vi "Bus Parameters to String.vi"(0 "Bus":T1={"Name"="", "Bus_Number"=0, "Bus_Controller"={"BC_Messages"=[{"Name"="Gun_One", "Tx-Rx_T-Tx"=FALSE, "RT_Address"=11, "RT_SA_Address"=10, "Parameters"=[{"name"="Data_01", "firstByte"=8, "startBit"=0, "numberBits"=8, "scaleFactor"=1.0, "scaleOffset"=0.0, "signed"=FALSE}], "Transfer Enabled"=TRUE, "Message Buffer ID"=0, "Default_Message_Buffer_Data"=[0, 1, 2, 3, 4, 5, 6, 7, 8, 9, 10, 11, 12, 13, 14, 15, 16, 17, 18, 19, 20, 21, 22, 23, 24, 25, 26, 27, 28, 29], "Word_Count"=30}, {"Name"="Gun_Two", "Tx-Rx_T-Tx"=FALSE, "RT_Address"=11, "RT_SA_Address"=5, "Parameters"=[{"name"="Data_02", "firstByte"=8, "startBit"=0, "numberBits"=8, "scaleFactor"=1.0, "scaleOffset"=0.0, "signed"=FALSE}], "Transfer Enabled"=TRUE, "Message Buffer ID"=1, "Default_Message_Buffer_Data"=[0, 5, 10, 15, 20, 25, 30, 35, 40, 45, 50, 55, 60, 65, 70, 75, 80, 85, 90, 95, 100, 105, 110, 115, 120, 125, 130, 135, 140, 145], "Word_Count"=30}, {"Name"="Get_It", "Tx-Rx_T-Tx"=TRUE, "RT_Address"=5, "RT_SA_Address"=4, "Parameters"=[{"name"="Data_00", "firstByte"=1, "startBit"=0, "numberBits"=8, "scaleFactor"=1.0, "scaleOffset"=0.0, "signed"=FALSE}], "Transfer Enabled"=TRUE, "Message Buffer ID"=2, "Default_Message_Buffer_Data"=[0, 25, 50, 75, 100, 125, 150, 175, 200, 225, 250, 275, 300, 325, 350, 375, 400, 425, 450, 475, 500, 525, 550, 575, 600, 625, 650, 675, 700, 725], "Word_Count"=30}], "Acyclic_Frames"=[], "Enabled"=FALSE}, "Bus_Monitor"={"Name"="", "BM_Messages"=[{"RT_Address"=5, "RT_SubAddress"=1, "Tx-Rx_T-Tx"=TRUE, "Parameters"=[], "Name"=""}, {"RT_Address"=5, "RT_SubAddress"=2, "Tx-Rx_T-Tx"=TRUE, "Parameters"=[], "Name"=""}, {"RT_Address"=5, "RT_SubAddress"=3, "Tx-Rx_T-Tx"=TRUE, "Parameters"=[], "Name"=""}, {"RT_Address"=5, "RT_SubAddress"=4, "Tx-Rx_T-Tx"=TRUE, "Parameters"=[{"name"="BM_Data_Parm_1", "firstByte"=1, "startBit"=0, "numberBits"=8, "scaleFactor"=1.0, "scaleOffset"=0.0, "signed"=FALSE}], "Name"=""}, {"RT_Address"=5, "RT_SubAddress"=5, "Tx-Rx_T-Tx"=TRUE, "Parameters"=[], "Name"=""}, {"RT_Address"=5, "RT_SubAddress"=6, "Tx-Rx_T-Tx"=TRUE, "Parameters"=[], "Name"=""}, {"RT_Address"=5, "RT_SubAddress"=7, "Tx-Rx_T-Tx"=TRUE, "Parameters"=[], "Name"=""}, {"RT_Address"=5, "RT_SubAddress"=8, "Tx-Rx_T-Tx"=TRUE, "Parameters"=[], "Name"=""}, {"RT_Address"=5, "RT_SubAddress"=9, "Tx-Rx_T-Tx"=TRUE, "Parameters"=[], "Name"=""}, {"RT_Address"=5, "RT_SubAddress"=10, "Tx-Rx_T-Tx"=TRUE, "Parameters"=[], "Name"=""}, {"RT_Address"=5, "RT_SubAddress"=11, "Tx-Rx_T-Tx"=TRUE, "Parameters"=[], "Name"=""}, {"RT_Address"=5, "RT_SubAddress"=12, "Tx-Rx_T-Tx"=TRUE, "Parameters"=[], "Name"=""}, {"RT_Address"=5, "RT_SubAddress"=13, "Tx-Rx_T-Tx"=TRUE, "Parameters"=[], "Name"=""}, {"RT_Address"=5, "RT_SubAddress"=14, "Tx-Rx_T-Tx"=TRUE, "Parameters"=[], "Name"=""}, {"RT_Address"=5, "RT_SubAddress"=15, "Tx-Rx_T-Tx"=TRUE, "Parameters"=[], "Name"=""}, {"RT_Address"=5, "RT_SubAddress"=16, "Tx-Rx_T-Tx"=TRUE, "Parameters"=[], "Name"=""}, {"RT_Address"=5, "RT_SubAddress"=17, "Tx-Rx_T-Tx"=TRUE, "Parameters"=[], "Name"=""}, {"RT_Address"=5, "RT_SubAddress"=18, "Tx-Rx_T-Tx"=TRUE, "Parameters"=[], "Name"=""}, {"RT_Address"=5, "RT_SubAddress"=19, "Tx-Rx_T-Tx"=TRUE, "Parameters"=[], "Name"=""}, {"RT_Address"=5, "RT_SubAddress"=20, "Tx-Rx_T-Tx"=TRUE, "Parameters"=[], "Name"=""}, {"RT_Address"=5, "RT_SubAddress"=21, "Tx-Rx_T-Tx"=TRUE, "Parameters"=[], "Name"=""}, {"RT_Address"=5, "RT_SubAddress"=22, "Tx-Rx_T-Tx"=TRUE, "Parameters"=[], "Name"=""}, {"RT_Address"=5, "RT_SubAddress"=23, "Tx-Rx_T-Tx"=TRUE, "Parameters"=[], "Name"=""}, {"RT_Address"=5, "RT_SubAddress"=24, "Tx-Rx_T-Tx"=TRUE, "Parameters"=[], "Name"=""}, {"RT_Address"=5, "RT_SubAddress"=25, "Tx-Rx_T-Tx"=TRUE, "Parameters"=[], "Name"=""}, {"RT_Address"=5, "RT_SubAddress"=26, "Tx-Rx_T-Tx"=TRUE, "Parameters"=[], "Name"=""}, {"RT_Address"=5, "RT_SubAddress"=27, "Tx-Rx_T-Tx"=TRUE, "Parameters"=[], "Name"=""}, {"RT_Address"=5, "RT_SubAddress"=28, "Tx-Rx_T-Tx"=TRUE, "Parameters"=[], "Name"=""}, {"RT_Address"=5, "RT_SubAddress"=29, "Tx-Rx_T-Tx"=TRUE, "Parameters"=[], "Name"=""}, {"RT_Address"=5, "RT_SubAddress"=30, "Tx-Rx_T-Tx"=TRUE, "Parameters"=[], "Name"=""}, {"RT_Address"=5, "RT_SubAddress"=31, "Tx-Rx_T-Tx"=TRUE, "Parameters"=[], "Name"=""}, {"RT_Address"=11, "RT_SubAddress"=1, "Tx-Rx_T-Tx"=TRUE, "Parameters"=[], "Name"=""}, {"RT_Address"=11, "RT_SubAddress"=2, "Tx-Rx_T-Tx"=TRUE, "Parameters"=[], "Name"=""}, {"RT_Address"=11, "RT_SubAddress"=3, "Tx-Rx_T-Tx"=TRUE, "Parameters"=[], "Name"=""}, {"RT_Address"=11, "RT_SubAddress"=4, "Tx-Rx_T-Tx"=TRUE, "Parameters"=[], "Name"=""}, {"RT_Address"=11, "RT_SubAddress"=5, "Tx-Rx_T-Tx"=TRUE, "Parameters"=[], "Name"=""}, {"RT_Address"=11, "RT_SubAddress"=6, "Tx-Rx_T-Tx"=TRUE, "Parameters"=[], "Name"=""}, {"RT_Address"=11, "RT_SubAddress"=7, "Tx-Rx_T-Tx"=TRUE, "Parameters"=[], "Name"=""}, {"RT_Address"=11, "RT_SubAddress"=8, "Tx-Rx_T-Tx"=TRUE, "Parameters"=[], "Name"=""}, {"RT_Address"=11, "RT_SubAddress"=9, "Tx-Rx_T-Tx"=TRUE, "Parameters"=[], "Name"=""}, {"RT_Address"=11, "RT_SubAddress"=10, "Tx-Rx_T-Tx"=TRUE, "Parameters"=[], "Name"=""}, {"RT_Address"=11, "RT_SubAddress"=11, "Tx-Rx_T-Tx"=TRUE, "Parameters"=[], "Name"=""}, {"RT_Address"=11, "RT_SubAddress"=12, "Tx-Rx_T-Tx"=TRUE, "Parameters"=[], "Name"=""}, {"RT_Address"=11, "RT_SubAddress"=13, "Tx-Rx_T-Tx"=TRUE, "Parameters"=[], "Name"=""}, {"RT_Address"=11, "RT_SubAddress"=14, "Tx-Rx_T-Tx"=TRUE, "Parameters"=[], "Name"=""}, {"RT_Address"=11, "RT_SubAddress"=15, "Tx-Rx_T-Tx"=TRUE, "Parameters"=[], "Name"=""}, {"RT_Address"=11, "RT_SubAddress"=16, "Tx-Rx_T-Tx"=TRUE, "Parameters"=[], "Name"=""}, {"RT_Address"=11, "RT_SubAddress"=17, "Tx-Rx_T-Tx"=TRUE, "Parameters"=[], "Name"=""}, {"RT_Address"=11, "RT_SubAddress"=18, "Tx-Rx_T-Tx"=TRUE, "Parameters"=[], "Name"=""}, {"RT_Address"=11, "RT_SubAddress"=19, "Tx-Rx_T-Tx"=TRUE, "Parameters"=[], "Name"=""}, {"RT_Address"=11, "RT_SubAddress"=20, "Tx-Rx_T-Tx"=TRUE, "Parameters"=[], "Name"=""}, {"RT_Address"=11, "RT_SubAddress"=21, "Tx-Rx_T-Tx"=TRUE, "Parameters"=[], "Name"=""}, {"RT_Address"=11, "RT_SubAddress"=22, "Tx-Rx_T-Tx"=TRUE, "Parameters"=[], "Name"=""}, {"RT_Address"=11, "RT_SubAddress"=23, "Tx-Rx_T-Tx"=TRUE, "Parameters"=[], "Name"=""}, {"RT_Address"=11, "RT_SubAddress"=24, "Tx-Rx_T-Tx"=TRUE, "Parameters"=[], "Name"=""}, {"RT_Address"=11, "RT_SubAddress"=25, "Tx-Rx_T-Tx"=TRUE, "Parameters"=[], "Name"=""}, {"RT_Address"=11, "RT_SubAddress"=26, "Tx-Rx_T-Tx"=TRUE, "Parameters"=[], "Name"=""}, {"RT_Address"=11, "RT_SubAddress"=27, "Tx-Rx_T-Tx"=TRUE, "Parameters"=[], "Name"=""}, {"RT_Address"=11, "RT_SubAddress"=28, "Tx-Rx_T-Tx"=TRUE, "Parameters"=[], "Name"=""}, {"RT_Address"=11, "RT_SubAddress"=29, "Tx-Rx_T-Tx"=TRUE, "Parameters"=[], "Name"=""}, {"RT_Address"=11, "RT_SubAddress"=30, "Tx-Rx_T-Tx"=TRUE, "Parameters"=[], "Name"=""}, {"RT_Address"=11, "RT_SubAddress"=31, "Tx-Rx_T-Tx"=TRUE, "Parameters"=[], "Name"=""}, {"RT_Address"=5, "RT_SubAddress"=1, "Tx-Rx_T-Tx"=FALSE, "Parameters"=[], "Name"=""}, {"RT_Address"=5, "RT_SubAddress"=2, "Tx-Rx_T-Tx"=FALSE, "Parameters"=[], "Name"=""}, {"RT_Address"=5, "RT_SubAddress"=3, "Tx-Rx_T-Tx"=FALSE, "Parameters"=[], "Name"=""}, {"RT_Address"=5, "RT_SubAddress"=4, "Tx-Rx_T-Tx"=FALSE, "Parameters"=[], "Name"=""}, {"RT_Address"=5, "RT_SubAddress"=5, "Tx-Rx_T-Tx"=FALSE, "Parameters"=[], "Name"=""}, {"RT_Address"=5, "RT_SubAddress"=6, "Tx-Rx_T-Tx"=FALSE, "Parameters"=[], "Name"=""}, {"RT_Address"=5, "RT_SubAddress"=7, "Tx-Rx_T-Tx"=FALSE, "Parameters"=[], "Name"=""}, {"RT_Address"=5, "RT_SubAddress"=8, "Tx-Rx_T-Tx"=FALSE, "Parameters"=[], "Name"=""}, {"RT_Address"=5, "RT_SubAddress"=9, "Tx-Rx_T-Tx"=FALSE, "Parameters"=[], "Name"=""}, {"RT_Address"=5, "RT_SubAddress"=10, "Tx-Rx_T-Tx"=FALSE, "Parameters"=[], "Name"=""}, {"RT_Address"=5, "RT_SubAddress"=11, "Tx-Rx_T-Tx"=FALSE, "Parameters"=[], "Name"=""}, {"RT_Address"=5, "RT_SubAddress"=12, "Tx-Rx_T-Tx"=FALSE, "Parameters"=[], "Name"=""}, {"RT_Address"=5, "RT_SubAddress"=13, "Tx-Rx_T-Tx"=FALSE, "Parameters"=[], "Name"=""}, {"RT_Address"=5, "RT_SubAddress"=14, "Tx-Rx_T-Tx"=FALSE, "Parameters"=[], "Name"=""}, {"RT_Address"=5, "RT_SubAddress"=15, "Tx-Rx_T-Tx"=FALSE, "Parameters"=[], "Name"=""}, {"RT_Address"=5, "RT_SubAddress"=16, "Tx-Rx_T-Tx"=FALSE, "Parameters"=[], "Name"=""}, {"RT_Address"=5, "RT_SubAddress"=17, "Tx-Rx_T-Tx"=FALSE, "Parameters"=[], "Name"=""}, {"RT_Address"=5, "RT_SubAddress"=18, "Tx-Rx_T-Tx"=FALSE, "Parameters"=[], "Name"=""}, {"RT_Address"=5, "RT_SubAddress"=19, "Tx-Rx_T-Tx"=FALSE, "Parameters"=[], "Name"=""}, {"RT_Address"=5, "RT_SubAddress"=20, "Tx-Rx_T-Tx"=FALSE, "Parameters"=[], "Name"=""}, {"RT_Address"=5, "RT_SubAddress"=21, "Tx-Rx_T-Tx"=FALSE, "Parameters"=[], "Name"=""}, {"RT_Address"=5, "RT_SubAddress"=22, "Tx-Rx_T-Tx"=FALSE, "Parameters"=[], "Name"=""}, {"RT_Address"=5, "RT_SubAddress"=23, "Tx-Rx_T-Tx"=FALSE, "Parameters"=[], "Name"=""}, {"RT_Address"=5, "RT_SubAddress"=24, "Tx-Rx_T-Tx"=FALSE, "Parameters"=[], "Name"=""}, {"RT_Address"=5, "RT_SubAddress"=25, "Tx-Rx_T-Tx"=FALSE, "Parameters"=[], "Name"=""}, {"RT_Address"=5, "RT_SubAddress"=26, "Tx-Rx_T-Tx"=FALSE, "Parameters"=[], "Name"=""}, {"RT_Address"=5, "RT_SubAddress"=27, "Tx-Rx_T-Tx"=FALSE, "Parameters"=[], "Name"=""}, {"RT_Address"=5, "RT_SubAddress"=28, "Tx-Rx_T-Tx"=FALSE, "Parameters"=[], "Name"=""}, {"RT_Address"=5, "RT_SubAddress"=29, "Tx-Rx_T-Tx"=FALSE, "Parameters"=[], "Name"=""}, {"RT_Address"=5, "RT_SubAddress"=30, "Tx-Rx_T-Tx"=FALSE, "Parameters"=[], "Name"=""}, {"RT_Address"=5, "RT_SubAddress"=31, "Tx-Rx_T-Tx"=FALSE, "Parameters"=[], "Name"=""}, {"RT_Address"=11, "RT_SubAddress"=1, "Tx-Rx_T-Tx"=FALSE, "Parameters"=[], "Name"=""}, {"RT_Address"=11, "RT_SubAddress"=2, "Tx-Rx_T-Tx"=FALSE, "Parameters"=[], "Name"=""}, {"RT_Address"=11, "RT_SubAddress"=3, "Tx-Rx_T-Tx"=FALSE, "Parameters"=[], "Name"=""}, {"RT_Address"=11, "RT_SubAddress"=4, "Tx-Rx_T-Tx"=FALSE, "Parameters"=[], "Name"=""}, {"RT_Address"=11, "RT_SubAddress"=5, "Tx-Rx_T-Tx"=FALSE, "Parameters"=[], "Name"=""}, {"RT_Address"=11, "RT_SubAddress"=6, "Tx-Rx_T-Tx"=FALSE, "Parameters"=[], "Name"=""}, {"RT_Address"=11, "RT_SubAddress"=7, "Tx-Rx_T-Tx"=FALSE, "Parameters"=[], "Name"=""}, {"RT_Address"=11, "RT_SubAddress"=8, "Tx-Rx_T-Tx"=FALSE, "Parameters"=[], "Name"=""}, {"RT_Address"=11, "RT_SubAddress"=9, "Tx-Rx_T-Tx"=FALSE, "Parameters"=[], "Name"=""}, {"RT_Address"=11, "RT_SubAddress"=10, "Tx-Rx_T-Tx"=FALSE, "Parameters"=[], "Name"=""}, {"RT_Address"=11, "RT_SubAddress"=11, "Tx-Rx_T-Tx"=FALSE, "Parameters"=[], "Name"=""}, {"RT_Address"=11, "RT_SubAddress"=12, "Tx-Rx_T-Tx"=FALSE, "Parameters"=[], "Name"=""}, {"RT_Address"=11, "RT_SubAddress"=13, "Tx-Rx_T-Tx"=FALSE, "Parameters"=[], "Name"=""}, {"RT_Address"=11, "RT_SubAddress"=14, "Tx-Rx_T-Tx"=FALSE, "Parameters"=[], "Name"=""}, {"RT_Address"=11, "RT_SubAddress"=15, "Tx-Rx_T-Tx"=FALSE, "Parameters"=[], "Name"=""}, {"RT_Address"=11, "RT_SubAddress"=16, "Tx-Rx_T-Tx"=FALSE, "Parameters"=[], "Name"=""}, {"RT_Address"=11, "RT_SubAddress"=17, "Tx-Rx_T-Tx"=FALSE, "Parameters"=[], "Name"=""}, {"RT_Address"=11, "RT_SubAddress"=18, "Tx-Rx_T-Tx"=FALSE, "Parameters"=[], "Name"=""}, {"RT_Address"=11, "RT_SubAddress"=19, "Tx-Rx_T-Tx"=FALSE, "Parameters"=[], "Name"=""}, {"RT_Address"=11, "RT_SubAddress"=20, "Tx-Rx_T-Tx"=FALSE, "Parameters"=[], "Name"=""}, {"RT_Address"=11, "RT_SubAddress"=21, "Tx-Rx_T-Tx"=FALSE, "Parameters"=[], "Name"=""}, {"RT_Address"=11, "RT_SubAddress"=22, "Tx-Rx_T-Tx"=FALSE, "Parameters"=[], "Name"=""}, {"RT_Address"=11, "RT_SubAddress"=23, "Tx-Rx_T-Tx"=FALSE, "Parameters"=[], "Name"=""}, {"RT_Address"=11, "RT_SubAddress"=24, "Tx-Rx_T-Tx"=FALSE, "Parameters"=[], "Name"=""}, {"RT_Address"=11, "RT_SubAddress"=25, "Tx-Rx_T-Tx"=FALSE, "Parameters"=[], "Name"=""}, {"RT_Address"=11, "RT_SubAddress"=26, "Tx-Rx_T-Tx"=FALSE, "Parameters"=[], "Name"=""}, {"RT_Address"=11, "RT_SubAddress"=27, "Tx-Rx_T-Tx"=FALSE, "Parameters"=[], "Name"=""}, {"RT_Address"=11, "RT_SubAddress"=28, "Tx-Rx_T-Tx"=FALSE, "Parameters"=[], "Name"=""}, {"RT_Address"=11, "RT_SubAddress"=29, "Tx-Rx_T-Tx"=FALSE, "Parameters"=[], "Name"=""}, {"RT_Address"=11, "RT_SubAddress"=30, "Tx-Rx_T-Tx"=FALSE, "Parameters"=[], "Name"=""}, {"RT_Address"=11, "RT_SubAddress"=31, "Tx-Rx_T-Tx"=FALSE, "Parameters"=[], "Name"=""}], "Address Set Inverted"=TRUE}, "RT_Messages"=[{"RT_Address"=5, "RT_SubAddress"=4, "Tx-Rx_T-Tx"=TRUE, "Parameters"=[{"name"="RT Data T", "firstByte"=1, "startBit"=0, "numberBits"=8, "scaleFactor"=1.0, "scaleOffset"=0.0, "signed"=FALSE}], "Message_Buffer ID"=0, "Default_Message_Buffer_Data"=[291, 292, 293, 0, 0, 0, 0, 273, 0, 0, 0, 0, 0, 0, 0, 0, 0, 0, 0, 0, 0, 0, 0, 0, 0, 0, 0, 0, 0, 0, 0, 0], "Word_Count"=32, "Name"=""}, {"RT_Address"=11, "RT_SubAddress"=5, "Tx-Rx_T-Tx"=TRUE, "Parameters"=[], "Message_Buffer ID"=0, "Default_Message_Buffer_Data"=[0, 0, 0, 0, 0, 0, 0, 0, 0, 0, 0, 0, 0, 0, 0, 0, 0, 0, 0, 0, 0, 0, 0, 0, 0, 0, 0, 0, 0, 0, 0, 0], "Word_Count"=32, "Name"=""}, {"RT_Address"=11, "RT_SubAddress"=10, "Tx-Rx_T-Tx"=TRUE, "Parameters"=[], "Message_Buffer ID"=0, "Default_Message_Buffer_Data"=[0, 0, 0, 0, 0, 0, 0, 0, 0, 0, 0, 0, 0, 0, 0, 0, 0, 0, 0, 0, 0, 0, 0, 0, 0, 0, 0, 0, 0, 0, 0, 0], "Word_Count"=32, "Name"=""}, {"RT_Address"=5, "RT_SubAddress"=4, "Tx-Rx_T-Tx"=FALSE, "Parameters"=[], "Message_Buffer ID"=0, "Default_Message_Buffer_Data"=[0, 0, 0, 0, 0, 0, 0, 0, 0, 0, 0, 0, 0, 0, 0, 0, 0, 0, 0, 0, 0, 0, 0, 0, 0, 0, 0, 0, 0, 0, 0, 0], "Word_Count"=32, "Name"=""}, {"RT_Address"=11, "RT_SubAddress"=5, "Tx-Rx_T-Tx"=FALSE, "Parameters"=[], "Message_Buffer ID"=0, "Default_Message_Buffer_Data"=[0, 0, 0, 0, 0, 0, 0, 0, 0, 0, 0, 0, 0, 0, 0, 0, 0, 0, 0, 0, 0, 0, 0, 0, 0, 0, 0, 0, 0, 0, 0, 0], "Word_Count"=32, "Name"=""}, {"RT_Address"=11, "RT_SubAddress"=10, "Tx-Rx_T-Tx"=FALSE, "Parameters"=[{"name"="RT Data R", "firstByte"=8, "startBit"=0, "numberBits"=8, "scaleFactor"=1.0, "scaleOffset"=0.0, "signed"=FALSE}], "Message_Buffer ID"=0, "Default_Message_Buffer_Data"=[0, 0, 0, 0, 0, 0, 0, 0, 0, 0, 0, 0, 0, 0, 0, 0, 0, 0, 0, 0, 0, 0, 0, 0, 0, 0, 0, 0, 0, 0, 0, 0], "Word_Count"=32, "Name"=""}]}) -> (4 "Parms List":string)   [LabVIEW 2013]
uses:
  Controls/1553_Bus.ctl
  Controls/1553_Bus_Controller.ctl
  Controls/1553_BC_Message.ctl
  Controls/664 -Param.ctl
  Controls/1553_Acyclic_Frame.ctl
  Controls/1553_Bus_Monitor.ctl
  Controls/1553_BM_Message.ctl
  Controls/1553_RT_Message.ctl
  AIT 664 Custom Device.lvlib
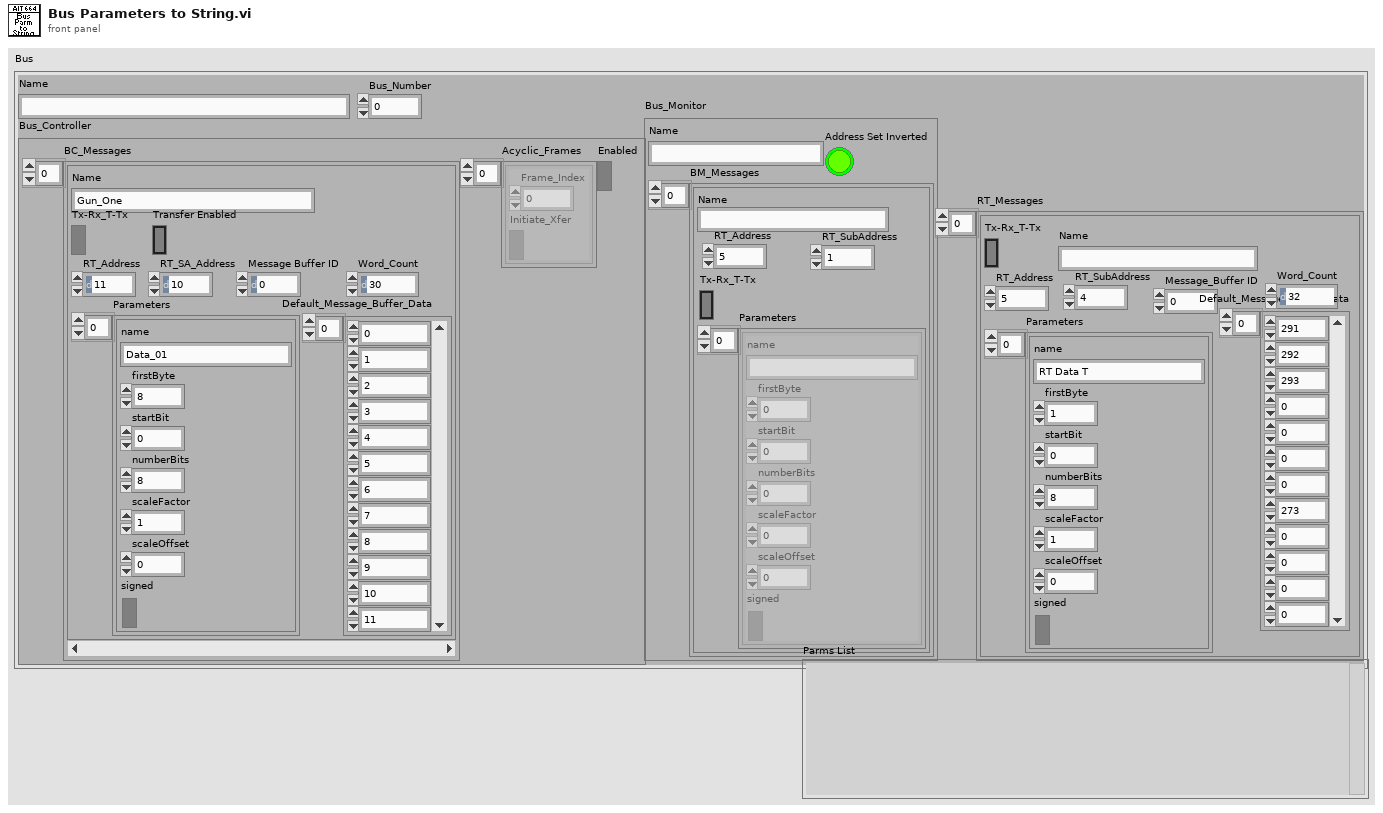
[diagram p1: front panel]
types:
  T1 = typedef "AIT 664 Custom Device.lvlib/1553_Bus.ctl" = cluster{"Name":string, "Bus_Number":u8, "Bus_Controller":T2, "Bus_Monitor":T6, "RT_Messages":T8[]}
  T2 = typedef "AIT 664 Custom Device.lvlib/1553_Bus_Controller.ctl" = cluster{"BC_Messages":T3[], "Acyclic_Frames":T5[], "Enabled":bool}
  T3 = typedef "AIT 664 Custom Device.lvlib/1553_BC_Message.ctl" = cluster{"Name":string, "Tx-Rx_T-Tx":bool, "RT_Address":u8, "RT_SA_Address":u8, "Parameters":T4[], "Transfer Enabled":bool, "Message Buffer ID":u16, "Default_Message_Buffer_Data":u16[], "Word_Count":u8}
  T4 = typedef "AIT 664 Custom Device.lvlib/664 -Param.ctl" = cluster{"name":string, "firstByte":i32, "startBit":i32, "numberBits":i32, "scaleFactor":dbl, "scaleOffset":dbl, "signed":bool}
  T5 = typedef "AIT 664 Custom Device.lvlib/1553_Acyclic_Frame.ctl" = cluster{"Frame_Index":u8, "Initiate_Xfer":bool}
  T6 = typedef "AIT 664 Custom Device.lvlib/1553_Bus_Monitor.ctl" = cluster{"Name":string, "BM_Messages":T7[], "Address Set Inverted":bool}
  T7 = typedef "AIT 664 Custom Device.lvlib/1553_BM_Message.ctl" = cluster{"RT_Address":u8, "RT_SubAddress":u8, "Tx-Rx_T-Tx":bool, "Parameters":T4[], "Name":string}
  T8 = typedef "AIT 664 Custom Device.lvlib/1553_RT_Message.ctl" = cluster{"RT_Address":u8, "RT_SubAddress":u8, "Tx-Rx_T-Tx":bool, "Parameters":T4[], "Message_Buffer ID":u16, "Default_Message_Buffer_Data":u16[], "Word_Count":u8, "Name":string}
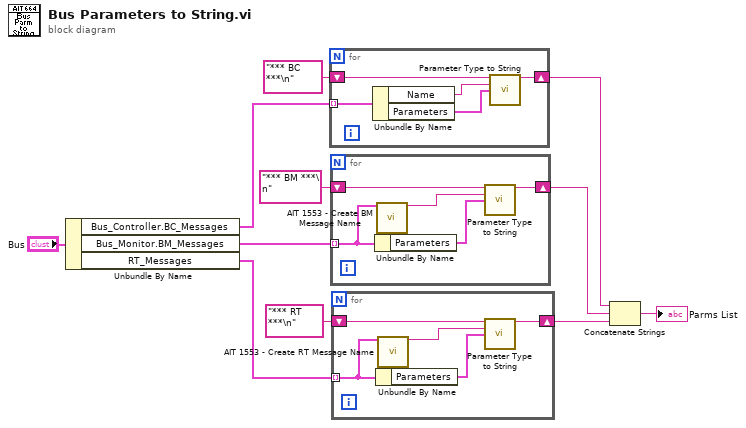
[diagram p0: block diagram]
diagram:
  n1 = Unbundle By Name("Bus") -> ("Bus_Controller.BC_Messages"=w10:T3[], "Bus_Monitor.BM_Messages"=w8:T7[], "RT_Messages"=w5:T8[])
  n2 = for {
    tunnel: w10 -> [w16] mode=indexing
    shift-right: [w15] -> w6
    shift-left: "*** BC ***\n" -> [w14]
    n3 = Unbundle By Name(w16) -> ("Name"=w12:string, "Parameters"=w13:T4[])
    n4 = call "Parameter Type to String.vi"("String in"=w14, "Message Name"=w12, "Parameters"=w13) -> ("String out"=w15:string)  [unwired: 12 in]
  }
  n5 = for {
    tunnel: w8 -> [w20] mode=indexing
    shift-right: [w21] -> w3
    shift-left: "*** BM ***\n" -> [w19]
    n6 = Unbundle By Name(w20) -> ("Parameters"=w17:T4[])
    n7 = call "AIT 1553 - Create BM Message Name.vi"("BM_Message"=w20) -> ("Message Name"=w18:string)  [unwired: 13 in, 1 out]
    n8 = call "Parameter Type to String.vi"("String in"=w19, "Message Name"=w18, "Parameters"=w17) -> ("String out"=w21:string)  [unwired: 12 in]
  }
  n9 = for {
    tunnel: w5 -> [w25] mode=indexing
    shift-right: [w26] -> w1
    shift-left: "*** RT ***\n" -> [w24]
    n10 = Unbundle By Name(w25) -> ("Parameters"=w22:T4[])
    n11 = call "AIT 1553 - Create RT Message Name.vi"("RT_Message"=w25) -> ("Message Name"=w23:string)  [unwired: 13 in, 1 out]
    n12 = call "Parameter Type to String.vi"("String in"=w24, "Message Name"=w23, "Parameters"=w22) -> ("String out"=w26:string)  [unwired: 12 in]
  }
  n13 = Concatenate Strings(w6, w3, w1) -> (→"Parms List":string)
